vi "logService_method_method_写入日志.vi"(4 "标志符号":string(combo)="LOGI", 6 "发生的所在的vi":string="未知", 8 "error in":errorcluster caption="错误输入（无错误）", 9 "内容":string="空", 10 "标题":string="无错误") -> (0 "error out":errorcluster caption="错误输出")   [LabVIEW 2014]
uses:
  R/manifest.vi
panel:
  # "年，月，日   小时：分钟：秒：   --标志符号--发生的所在的vi-标题： 消息内容"
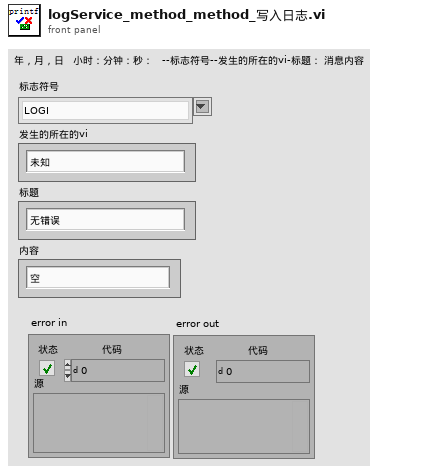
[diagram p1: front panel]
types:
  T1 = cluster{"标题":string, "相对路径":string, "类型":enum16{"服务", "活动"}, "专属队列名称":string}
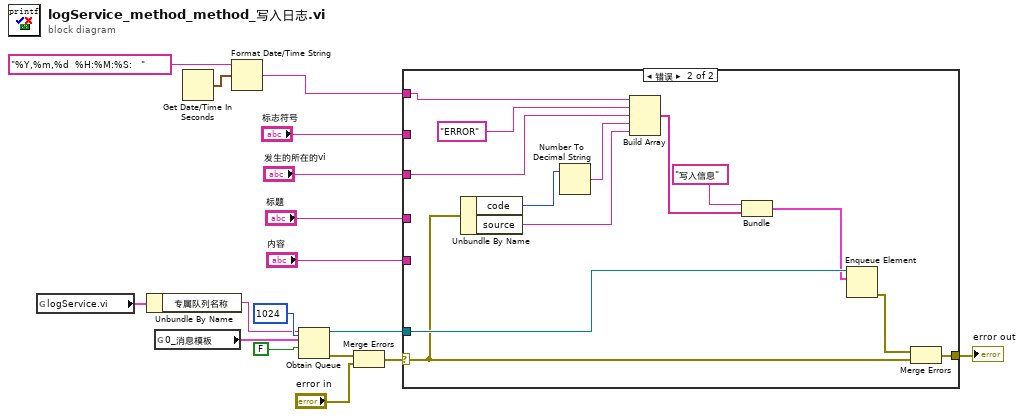
[diagram p0: block diagram]
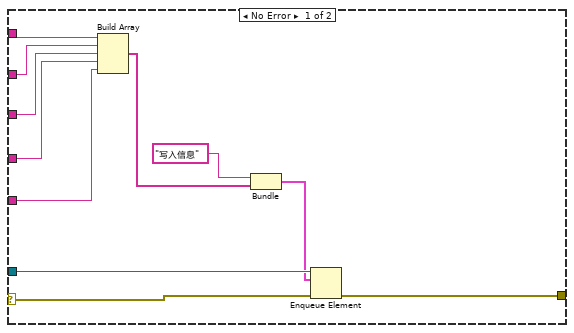
[diagram p2: hidden frame]
diagram:
  n1 = global read "manifest.vi" "logService.vi"() -> (w6:T1)
  n2 = Unbundle By Name(w6) -> ("专属队列名称"=w5:string)
  n3 = global read "manifest.vi" "0_消息模板"() -> (w9:cluster{"消息":string, "数据":variant})
  n4 = Get Date/Time In Seconds() -> (seconds since 1Jan1904=w16:timestamp)
  n5 = Format Date/Time String(time format string (%c)="%Y,%m,%d  %H:%M:%S:   " ("时间格式字符串(%c)"), seconds (now)=w16) -> (date/time string=w14:string)  [unwired: 1 in]
  n6 = Obtain Queue(max queue size (-1, unlimited)=1024 ("队列最大值（-1，无限）"), name (unnamed)=w5, element data type=w9, create if not found? (T)=FALSE ("如未找到是否创建？(T)")) -> (queue out=w1:refnum<queue>, error out=w3:errorcluster)  [unwired: 1 in, 1 out]
  n7 = Merge Errors(w3, "error in") -> (w2:errorcluster)
  n8 = case shown="错误" w2 {
    selector: w2 -> [w19 w30]
    tunnel: [w18 w31] -> w17
    tunnel: w1 -> [w28 w40]
    tunnel: w14 -> [w26 w39]
    tunnel: "标志符号" -> [w25 _]
    tunnel: "发生的所在的vi" -> [w24 w37]
    tunnel: "标题" -> [w23 _]
    tunnel: "内容" -> [w22 _]
    frame No Error {
      n9 = Build Array(w26, w25, w24, w23, w22) -> (w21:string[])
      n10 = Bundle("字符串"="写入信息", w21) -> (w20:cluster{"字符串":string, string[]})  [unwired: 1 in]
      n11 = Enqueue Element(queue=w28, element=w20, error in (no error)=w19) -> (error out=w18:errorcluster)  [unwired: 1 in, 2 out]
    }
    frame Error {
      n12 = Unbundle By Name(w30) -> ("code"=w41:i32, "source"=w35:string)
      n13 = Number To Decimal String(number=w41) -> (decimal integer string=w36:string)  [unwired: 1 in]
      n14 = Build Array(w39, "ERROR" ("字符串"), w37, w36, w35) -> (w33:string[])
      n15 = Bundle("字符串"="写入信息", w33) -> (w32:cluster{"字符串":string, string[]})  [unwired: 1 in]
      n16 = Enqueue Element(queue=w40, element=w32) -> (error out=w29:errorcluster)  [unwired: 2 in, 2 out]
      n17 = Merge Errors(w29, w30) -> (w31:errorcluster)
    }
  }
  "error out" <- w17
